vi "生成手机号码数据.vi"(11 "字符串":string) -> (3 "手机号码内容":u8[](array[numeric]) format="%x")   [LabVIEW 2015]
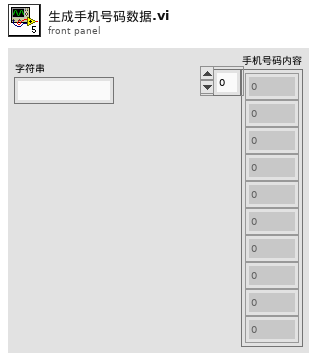
[diagram p1: front panel]
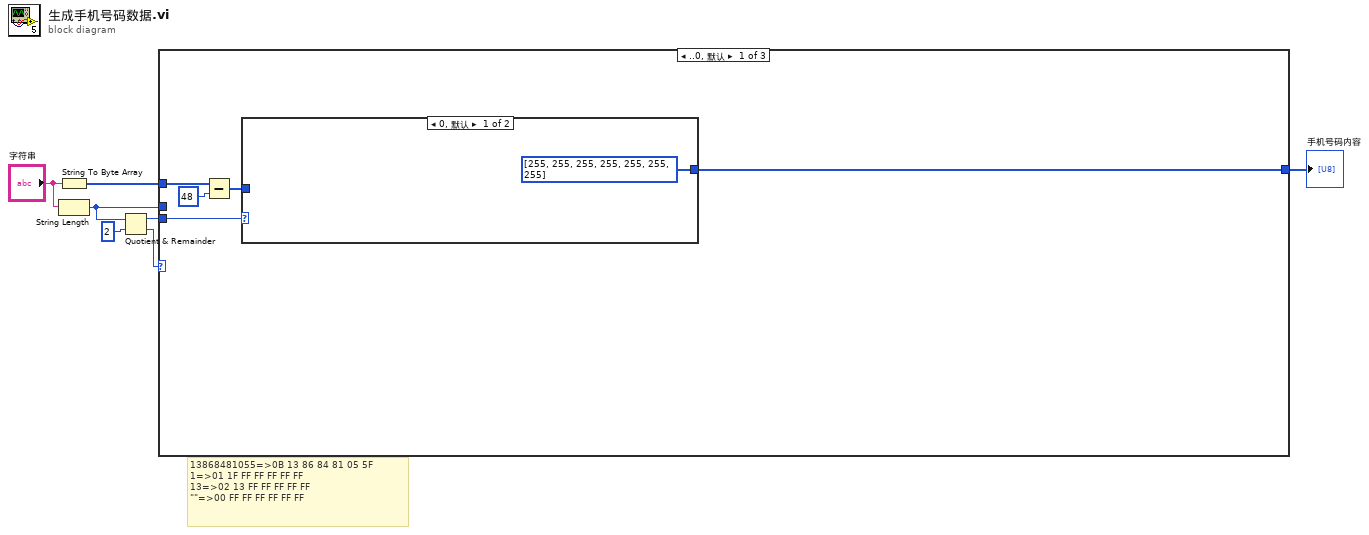
[diagram p0: block diagram]
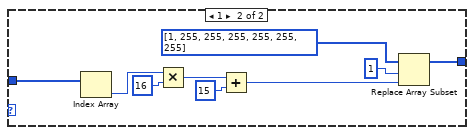
[diagram p2: hidden frame]
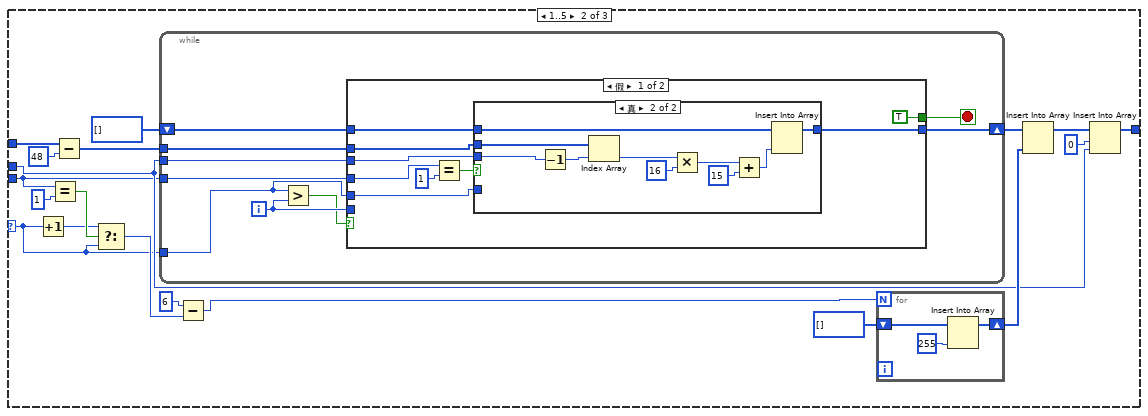
[diagram p3: hidden frame]
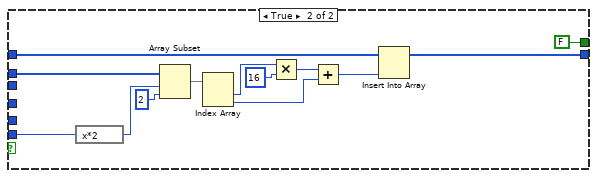
[diagram p5: hidden frame]
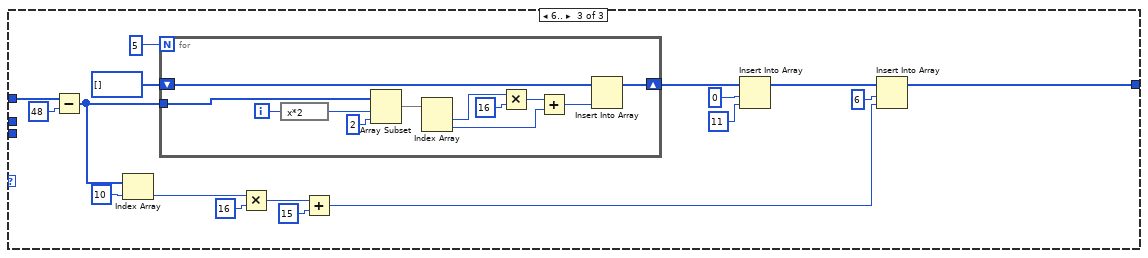
[diagram p6: hidden frame]
diagram:
  # "13868481055=>0B 13 86 84 81 05 5F\n1=>01 1F FF FF FF FF FF\n13=>02 13 FF FF FF FF FF\n\"\"=>00 FF FF FF FF FF FF"
  n1 = String To Byte Array(string="字符串") -> (unsigned byte array=w5:u8[])
  n2 = String Length(string="字符串") -> (length=w1:i32)
  n3 = Quotient & Remainder(x=w1, y=2) -> (x-y*floor(x/y)=w2:i32, floor(x/y)=w3:i32)
  n4 = case shown="..0, 默认" w3 {
    selector: w3 -> [_ w23 _]
    tunnel: [w11 w31 w95] -> w6
    tunnel: w5 -> [w9 w40 w97]
    tunnel: w2 -> [w12 w28 _]
    tunnel: w1 -> [_ w29 _]
    frame ..0, Default {
      n5 = Subtract(x=w9, y=u8 48) -> (x-y=w8:u8[])
      n6 = case shown="0, 默认" w12 {
        tunnel: [u8[] [255, 255, 255, 255, 255, 255, 255] w16] -> w11
        tunnel: w8 -> [_ w22]
        frame 0, Default {
        }
        frame 1 {
          n7 = Index Array(array=w22) -> (element=w21:u8)  [unwired: 1 in]
          n8 = Multiply(x=w21, y=u8 16) -> (x*y=w19:u8)
          n9 = Add(x=w19, y=u8 15) -> (x+y=w14:u8)
          n10 = Replace Array Subset(array=u8[] [1, 255, 255, 255, 255, 255, 255], new element=w14, index=1 ("索引")) -> (w16:u8[])
        }
      }
    }
    frame 1..5 {
      n11 = Increment(x=w23) -> (x+1=w24:i32)
      n12 = Equal?(x=w28, y=1) -> (x = y?=w26:bool)
      n13 = Subtract(x=w40, y=u8 48) -> (x-y=w39:u8[])
      n14 = Select(t=w24, s=w26, f=w23) -> (s? t:f=w25:i32)
      n15 = while {
        tunnel: w39 -> [w53]
        shift-right: [w51] -> w35
        shift-left: u8[] [] -> [w50]
        tunnel: w28 -> [w47]
        tunnel: w23 -> [w45]
        tunnel: w29 -> [w46]
        i -> [w49]
        stop <- w52 stop-if-true
        n16 = Greater?(x=w45, y=w49) -> (0:w48:bool)
        n17 = case shown="假" w48 {
          tunnel: w53 -> [w58 w86]
          tunnel: [TRUE FALSE] -> w52
          tunnel: [w56 w77] -> w51
          tunnel: w50 -> [w57 w76]
          tunnel: w49 -> [_ w75]
          tunnel: w47 -> [w62 _]
          tunnel: w46 -> [w55 _]
          tunnel: w45 -> [w54 _]
          frame False {
            n18 = Equal?(x=w62, y=1) -> (x = y?=w60:bool)
            n19 = case shown="真" w60 {
              tunnel: w58 -> [_ w70]
              tunnel: w57 -> [w63 w68]
              tunnel: [w63 w67] -> w56
              tunnel: w55 -> [_ w65]
              tunnel: w54 -> [_ _]
              frame False {
              }
              frame True {
                n20 = Decrement(x=w65) -> (x-1=w64:i32)
                n21 = Index Array(array=w70, index=w64) -> (element=w71:u8)
                n22 = Multiply(x=w71, y=u8 16) -> (x*y=w72:u8)
                n23 = Add(x=w72, y=u8 15) -> (x+y=w66:u8)
                n24 = Insert Into Array(array=w68, new element=w66) -> (w67:u8[])  [unwired: 1 in]
              }
            }
          }
          frame True {
            n25 = expression code="x*2"(w75) -> (w83:i32)
            n26 = Array Subset(array=w86, index=w83, length=2 ("长度")) -> (w84:u8[])
            n27 = Index Array(array=w84) -> (element #1=w81:u8, element #2=w80:u8)  [unwired: 2 in]
            n28 = Multiply(x=w81, y=u8 16) -> (x*y=w79:u8)
            n29 = Add(x=w79, y=w80) -> (x+y=w78:u8)
            n30 = Insert Into Array(array=w76, new element=w78) -> (w77:u8[])  [unwired: 1 in]
          }
        }
      }
      n31 = Subtract(x=6, y=w25) -> (x-y=w36:i32)
      n32 = for {
        N: w36 -> [_]
        shift-right: [w43] -> w34
        shift-left: u8[] [] -> [w44]
        n33 = Insert Into Array(array=w44, new element=u8 255 ("新元素/子数组")) -> (w43:u8[])  [unwired: 1 in]
      }
      n34 = Insert Into Array(array=w35, new element=w34) -> (w30:u8[])  [unwired: 1 in]
      n35 = Insert Into Array(array=w30, index=0 ("索引"), new element=w29) -> (w31:u8[])
    }
    frame 6.. {
      n36 = Subtract(x=w97, y=u8 48) -> (x-y=w88:u8[])
      n37 = Index Array(array=w88, index=10 ("索引")) -> (element=w91:u8)
      n38 = for {
        N: 5 -> [_]
        tunnel: w88 -> [w115]
        shift-right: [w105] -> w99
        shift-left: u8[] [] -> [w104]
        i -> [w112]
        n39 = expression code="x*2"(w112) -> (w111:i32)
        n40 = Array Subset(array=w115, index=w111, length=2 ("长度")) -> (w113:u8[])
        n41 = Index Array(array=w113) -> (element #1=w109:u8, element #2=w108:u8)  [unwired: 2 in]
        n42 = Multiply(x=w109, y=u8 16) -> (x*y=w107:u8)
        n43 = Add(x=w107, y=w108) -> (x+y=w106:u8)
        n44 = Insert Into Array(array=w104, new element=w106) -> (w105:u8[])  [unwired: 1 in]
      }
      n45 = Multiply(x=w91, y=u8 16) -> (x*y=w92:u8)
      n46 = Add(x=w92, y=u8 15) -> (x+y=w90:u8)
      n47 = Insert Into Array(array=w99, index=0 ("索引"), new element=u8 11 ("新元素/子数组")) -> (w96:u8[])
      n48 = Insert Into Array(array=w96, index=6 ("索引"), new element=w90) -> (w95:u8[])
    }
  }
  "手机号码内容" <- w6
